vi "WPI_RobotDriveMotors2.vi"(8 "error in (no error)":errorcluster, 9 "RightSpeed":dbl, 10 "LeftSpeed":dbl, 11 "RobotDriveDevRef":T1={"DevStatus"={"status"=FALSE, "code"=0, "source"=""}, "Motors[]"=[], "Square Inputs"=FALSE, "Max Output"=1.0, "Isochronous"=FALSE}) -> (0 "error out":errorcluster, 3 "RobotDriveDevRef":T1={"DevStatus"={"status"=FALSE, "code"=0, "source"=""}, "Motors[]"=[], "Square Inputs"=FALSE, "Max Output"=1.0, "Isochronous"=FALSE})   [LabVIEW 2011]
doc: "Determines the motor configuration and sends the speed values to the appropriate motors.\n\nThis software is licensed. Open the labview\\readme\\WPI Robotics Library Open Source License.txt file for more information."
uses:
  <vilib>/Rock Robotics/WPI/RobotDrive/WPI_RobotDriveDevRef.ctl
  <vilib>/Rock Robotics/WPI/MotorControl/WPI_MotorControlDeviceRef.ctl
  <vilib>/Rock Robotics/SystemInterfaces/Typedef/FPGA_TypedefDigitalModule.ctl
  <vilib>/Rock Robotics/SystemInterfaces/DIO/FPGA_DIOPWMChannel.ctl
  <vilib>/Rock Robotics/WPI/PWM/WPI_PWMDeadband.ctl
  <vilib>/Rock Robotics/WPI/CAN/Jaguar/SubVIs/WPI_CANJaguar_ControlMode.ctl
  <vilib>/Rock Robotics/WPI/PWM/WPI_PWMTransform_ConPane.ctl
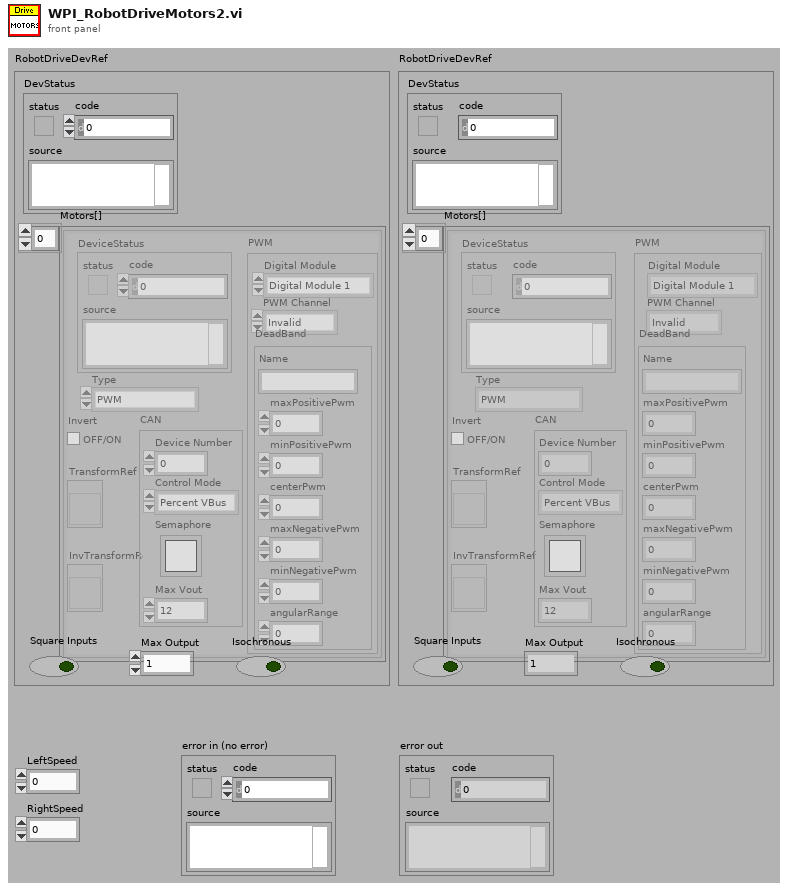
[diagram p1: front panel]
types:
  T1 = typedef "WPI_RobotDriveDevRef.ctl" = cluster{"DevStatus":errorcluster, "Motors[]":T2[], "Square Inputs":bool, "Max Output":dbl, "Isochronous":bool}
  T2 = typedef "WPI_MotorControlDeviceRef.ctl" = cluster{"DeviceStatus":errorcluster, "Type":enum16{"PWM", "CAN"}, "PWM":cluster{"Digital Module":T3, "PWM Channel":T4, "DeadBand":T5}, "CAN":cluster{"Device Number":u8, "Control Mode":T6, "Semaphore":T7, "Max Vout":dbl}, "Invert":bool, "TransformRef":T8, "InvTransformRef":T8}
  T3 = typedef "FPGA_TypedefDigitalModule.ctl" = enum16{"Digital Module 1", "Digital Module 2"}
  T4 = typedef "FPGA_DIOPWMChannel.ctl" = enum8{"PWM 1", "PWM 2", "PWM 3", "PWM 4", "PWM 5", "PWM 6", "PWM 7", "PWM 8", "PWM 9", "PWM 10", "Invalid"}
  T5 = typedef "WPI_PWMDeadband.ctl" = cluster{"Name":string, "maxPositivePwm":i32, "minPositivePwm":i32, "centerPwm":i32, "maxNegativePwm":i32, "minNegativePwm":i32, "angularRange":u16}
  T6 = typedef "WPI_CANJaguar_ControlMode.ctl" = enum8{"Percent VBus", "Current", "Speed", "Position", "Voltage"}
  T7 = typedef "Semaphore RefNum" = refnum<k1>
  T8 = typedef "WPI_PWMTransform_ConPane.ctl" = refnum<vi>
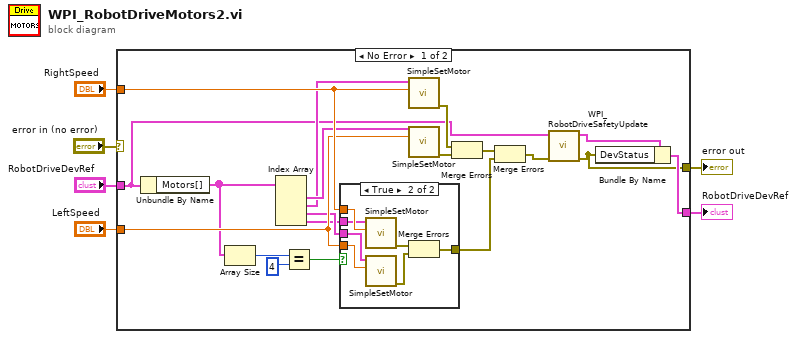
[diagram p0: block diagram]
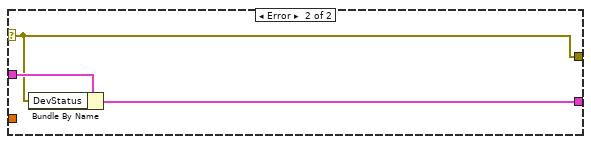
[diagram p3: hidden frame]
diagram:
  n1 = case shown="No Error" "error in (no error)" {
    selector: "error in (no error)" -> [_ w34]
    tunnel: "RobotDriveDevRef" -> [w9 w35]
    tunnel: [w23 w33] -> w5
    tunnel: "LeftSpeed" -> [w21 _]
    tunnel: "RightSpeed" -> [w22 _]
    tunnel: [w7 w34] -> w1
    frame No Error {
      n2 = Unbundle By Name(w9) -> ("Motors[]"=w15:T2[])
      n3 = Array Size(array=w15) -> (size(s)=w25:i32)
      n4 = Index Array(array=w15) -> (element #1=w14:T2, element #2=w13:T2, element #3=w12:T2, element #4=w11:T2)  [unwired: 4 in]
      n5 = Equal?(x=w25, y=4) -> (x = y?=w18:bool)
      n6 = case shown="True" w18 {
        tunnel: w22 -> [_ w32]
        tunnel: w21 -> [_ w31]
        tunnel: [_ w28] -> w17
        tunnel: w12 -> [_ w27]
        tunnel: w11 -> [_ w26]
        frame False {
        }
        frame True {
          n7 = call "SimpleSetMotor.vi"("Output"=w32, "MotorControlDevRef"=w26) -> ("error out"=w30:errorcluster)  [unwired: 8 in, 1 out]
          n8 = call "SimpleSetMotor.vi"("Output"=w31, "MotorControlDevRef"=w27) -> ("error out"=w29:errorcluster)  [unwired: 8 in, 1 out]
          n9 = Merge Errors(w30, w29) -> (w28:errorcluster)
        }
      }
      n10 = call "SimpleSetMotor.vi"("Output"=w22, "MotorControlDevRef"=w13) -> ("error out"=w20:errorcluster)  [unwired: 8 in, 1 out]
      n11 = call "SimpleSetMotor.vi"("Output"=w21, "MotorControlDevRef"=w14) -> ("error out"=w19:errorcluster)  [unwired: 8 in, 1 out]
      n12 = Merge Errors(w20, w19) -> (w16:errorcluster)
      n13 = Merge Errors(w16, w17) -> (w8:errorcluster)
      n14 = call <vilib>:"WPI_RobotDriveSafetyUpdate.vi"("error in (no error)"=w8, "RobotDriveDevRef"=w9) -> ("error out"=w7:errorcluster, "RobotDriveDevRef"=w10:T1)  [unwired: 8 out]
      n15 = Bundle By Name(cluster=w10, "DevStatus"=w7) -> (w23:T1)
    }
    frame Error {
      n16 = Bundle By Name(cluster=w35, "DevStatus"=w34) -> (w33:T1)
    }
  }
  "RobotDriveDevRef" <- w5
  "error out" <- w1
